vi "Read config file data.vi"(8 "error in (no error)":errorcluster, 10 "Config In":variant, 11 "Turret in":refnum<class "Turret.lvclass">) -> (0 "error out":errorcluster, 3 "Turret out":refnum<class "Turret.lvclass">)   [LabVIEW 2019, in "Turret.lvlib" / "Turret.lvclass"]
uses:
  Turret.lvclass
  <vilib>/Rock Robotics/SystemInterfaces/AI/FPGA_AIChannel.ctl
  Turret.lvclass/Turret.ctl
  fec586d1-1d2f-4d3f-9967-f2aef551462b.vi
  75a0495f-ead6-4612-9604-30b4c119aa4f.vi
  34c177d3-23f6-4020-a247-071641e4add4.vi
  1038a51f-6de5-430d-a821-b7846f654ad2.vi
  <vilib>/Utility/error.llb/Trim Whitespace.vi
  <vilib>/Utility/error.llb/Error Cluster From Error Code.vi
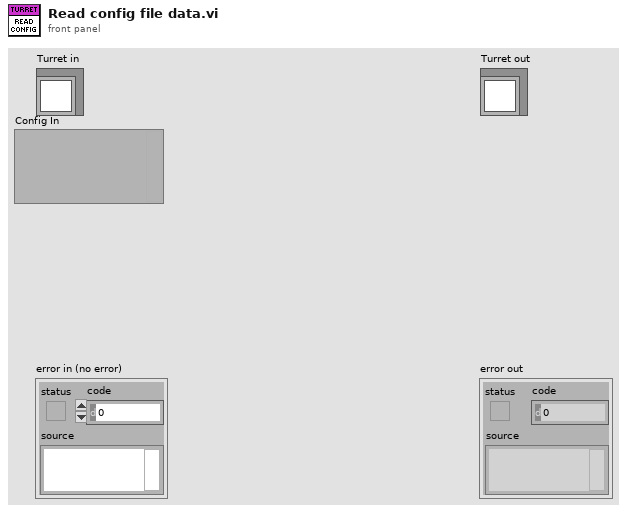
[diagram p1: front panel]
types:
  T1 = cluster{"proportional gain (Kc)":dbl, "integral time (Ti, min)":dbl, "derivative time (Td, min)":dbl}
  T2 = typedef "FPGA_AIChannel.ctl" = enum8{"AI 0", "AI 1", "AI 2", "AI 3", "AI MXP 0", "AI MXP 1", "AI MXP 2", "AI MXP 3", "Invalid"}
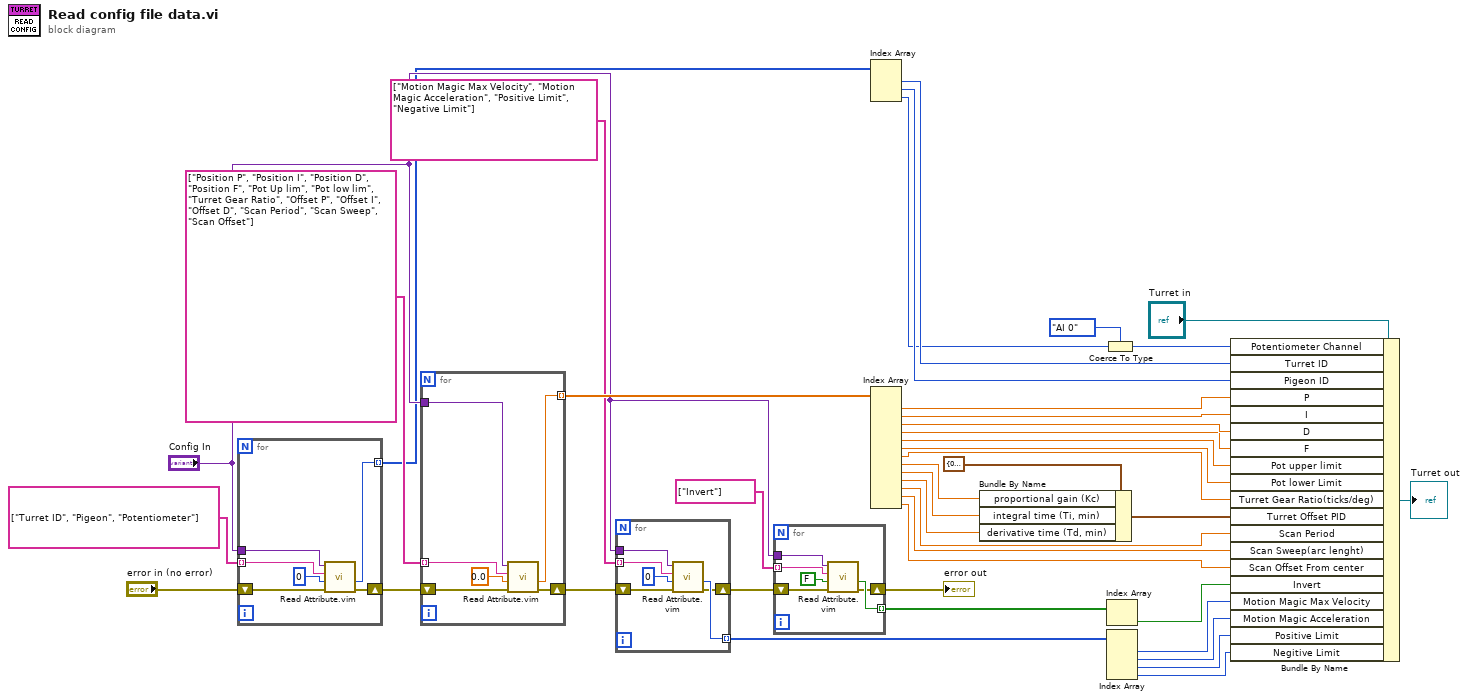
[diagram p0: block diagram]
diagram:
  n1 = for {
    tunnel: "Config In" -> [w47]
    tunnel: string[] ["Turret ID", "Pigeon", "Potentiometer"] -> [w46] mode=indexing
    tunnel: [w45] -> w31 mode=indexing
    shift-right: [w43] -> w26
    shift-left: "error in (no error)" -> [w44]
    n2 = call "Read Attribute.vim"("error in"=w44, "default value (data type)"=u8 0, "name"=w46, "variant in"=w47) -> ("error out"=w43:errorcluster, "value"=w45:u8)  [unwired: 4 in, 2 out]
  }
  n3 = for {
    tunnel: "Config In" -> [w53]
    tunnel: string[] ["Position P", "Position I", "Position D", "Position F", "Pot Up lim", "Pot low lim", "Turret Gear Ratio", "Offset P", "Offset I", "Offset D", "Scan Period", "Scan Sweep", "Scan Offset"] -> [w52] mode=indexing
    tunnel: [w50] -> w40 mode=indexing
    shift-right: [w48] -> w25
    shift-left: w26 -> [w49]
    n4 = call "Read Attribute.vim"("error in"=w49, "default value (data type)"=0.0, "name"=w52, "variant in"=w53) -> ("error out"=w48:errorcluster, "value"=w50:dbl)  [unwired: 4 in, 2 out]
  }
  n5 = for {
    tunnel: "Config In" -> [w59]
    tunnel: [w58] -> w33 mode=indexing
    shift-right: [w56] -> w24
    shift-left: w25 -> [w57]
    tunnel: string[] ["Motion Magic Max Velocity", "Motion Magic Acceleration", "Positive Limit", "Negative Limit"] -> [w54] mode=indexing
    n6 = call "Read Attribute.vim"("error in"=w57, "default value (data type)"=0, "name"=w54, "variant in"=w59) -> ("error out"=w56:errorcluster, "value"=w58:i32)  [unwired: 4 in, 2 out]
  }
  n7 = for {
    tunnel: "Config In" -> [w65]
    tunnel: string[] ["Invert"] -> [w64] mode=indexing
    tunnel: [w63] -> w34 mode=indexing
    shift-right: [w61] -> w23
    shift-left: w24 -> [w62]
    n8 = call "Read Attribute.vim"("error in"=w62, "default value (data type)"=FALSE, "name"=w64, "variant in"=w65) -> ("error out"=w61:errorcluster, "value"=w63:bool)  [unwired: 4 in, 2 out]
  }
  "error out" <- w23
  n9 = Index Array(array=w31) -> (element #1=w30:u8, element #2=w29:u8, element #3=w28:u8)  [unwired: 3 in]
  n10 = Index Array(array=w40) -> (element #1=w22:dbl, element #2=w21:dbl, element #3=w20:dbl, element #4=w19:dbl, element #5=w14:dbl, element #6=w13:dbl, element #7=w12:dbl, element #8=w8:dbl, element #9=w7:dbl, element #10=w6:dbl, element #11=w5:dbl, element #12=w4:dbl, element #13=w3:dbl)  [unwired: 13 in]
  n11 = Bundle By Name(cluster=T1 {"proportional gain (Kc)"=0.0, "integral time (Ti, min)"=0.0, "derivative time (Td, min)"=0.0} ("Turret Offset PID"), "proportional gain (Kc)"=w8, "integral time (Ti, min)"=w7, "derivative time (Td, min)"=w6) -> (w10:T1)
  n12 = Coerce To Type(0:w28, 1:FPGA_AIChannel."AI 0" ("Potentiometer Channel")) -> (2:w18:T2)
  n13 = Index Array(array=w34) -> (element=w9:bool)  [unwired: 1 in]
  n14 = Index Array(array=w33) -> (element #1=w17:i32, element #2=w16:i32, element #3=w2:i32, element #4=w1:i32)  [unwired: 4 in]
  n15 = Bundle By Name(cluster="Turret in", "Potentiometer Channel"=w18, "Turret ID"=w30, "Pigeon ID"=w29, "P"=w22, "I"=w21, "D"=w20, "F"=w19, "Pot upper limit"=w14, "Pot lower Limit"=w13, "Turret Gear Ratio(ticks/deg)"=w12, "Turret Offset PID"=w10, "Scan Period"=w5, "Scan Sweep(arc lenght)"=w4, "Scan Offset From center"=w3, "Invert"=w9, "Motion Magic Max Velocity"=w17, "Motion Magic Acceleration"=w16, "Positive Limit"=w2, "Negitive Limit"=w1) -> (→"Turret out":refnum<class "Turret.lvclass">)
